vi "ReadWrite.Data.Buffer.vi"(8 "error in":errorcluster, 9 "Offset":i32, 10 "Values":dbl[](array[numeric]), 11 "Ref":T1) -> (0 "error out":errorcluster)   [LabVIEW 2024, in "VS Plugin Inline Async API.lvlib" / "Plugin Data Access.lvclass"]
uses:
  Plugin Data Access.lvclass
  Plugin Data Access.lvclass/Plugin Data Access.ctl
  ReadWrite/ReadWrite.lvclass
  ReadWrite.DVR.ctl
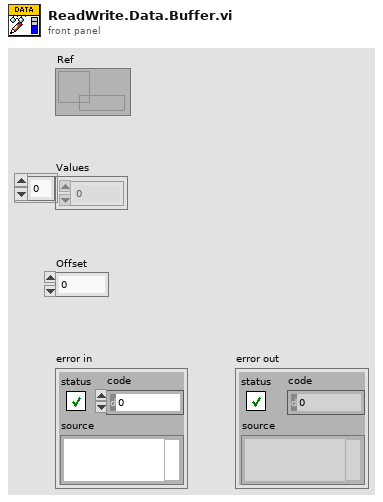
[diagram p1: front panel]
types:
  T1 = typedef "VS Plugin Inline Async API.lvlib/Plugin Data Access.lvclass/ReadWrite.DVR.ctl" = refnum<data-value>
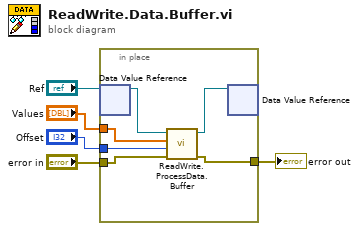
[diagram p0: block diagram]
diagram:
  n1 = in-place {
    in-place-border: "error in" -> [w10]
    in-place-border: "Values" -> [w7]
    in-place-border: "Offset" -> [w6]
    in-place-border: [w11] -> w4
    n2 = in-place-dvr #1("Ref") -> (w9:refnum<class "ReadWrite.lvclass">)  [unwired: 1 out]
    n3 = call "ReadWrite.ProcessData.Buffer.vi"("error in"=w10, "Offset"=w6, "Values"=w7, "ReadWrite in"=w9) -> ("error out"=w11:errorcluster, "ReadWrite out"=w8:refnum<class "ReadWrite.lvclass">)  [unwired: 6 in]
    n4 = in-place-dvr #1(w8) -> ()  [unwired: 2 out]
  }
  "error out" <- w4
